vi "Add Subscription.vi"(6 "Notification?(F)":bool, 8 "error in (no error)":errorcluster, 9 "Service Type":T1=4 items=["ONCE_ONLY"=1, "TIMED"=2, "MONITORED"=4], 10 "Subscription Name":string, 11 "DIMActor in":refnum<class "DIMActor.lvclass">) -> (0 "error out":errorcluster, 3 "DIMActor out":refnum<class "DIMActor.lvclass">)   [LabVIEW 2012, in "DIMActor.lvlib" / "DIMActor.lvclass"]
doc: "Subscribe to a DIM service."
uses:
  DIMActor.lvclass
  SVN/LV2009/GPL/lib.lib/DimLVEvent/LVDimInterface/LVDimInterface.dim service type.ctl
  DIMActor.lvclass/DIMActor.ctl
  SVN/LV2009/GPL/lib.lib/DimLVEvent/LVDimInterface/LVDimInterface.dic_info_service_notifier.vi
  SVN/LV2009/GPL/lib.lib/DimLVEvent/LVDimInterface/LVDimInterface.dic_info_service_queue.vi
  SVN/LV2009/GPL/lib.lib/DimLVEvent/LVDimInterface/LVDimInterface.lvlib
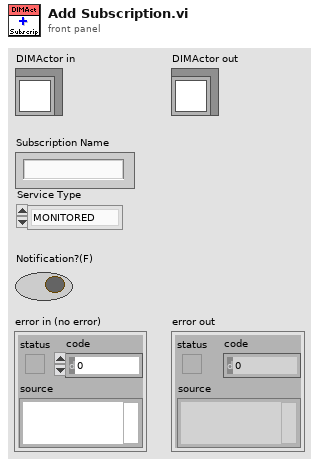
[diagram p1: front panel]
types:
  T1 = typedef "LVDimInterface.lvlib/LVDimInterface.dim service type.ctl" = u16
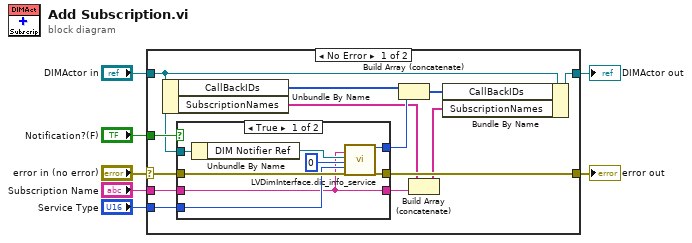
[diagram p0: block diagram]
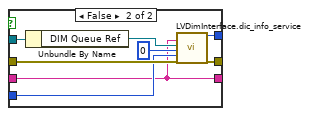
[diagram p2: hidden frame]
diagram:
  n1 = case shown="No Error" "error in (no error)" {
    selector: "error in (no error)" -> [w20 w38]
    tunnel: [w19 w38] -> w6
    tunnel: [w12 w37] -> w4
    tunnel: "DIMActor in" -> [w13 w37]
    tunnel: "Subscription Name" -> [w18 _]
    tunnel: "Notification?(F)" -> [w14 _]
    tunnel: "Service Type" -> [w8 _]
    frame No Error {
      n2 = Unbundle By Name(w13) -> ("CallBackIDs"=w15:i32[], "SubscriptionNames"=w11:string[])
      n3 = case shown="True" w14 {
        tunnel: w20 -> [w25 w33]
        tunnel: [w24 w32] -> w19
        tunnel: w18 -> [w21 w29]
        tunnel: [w26 w34] -> w17
        tunnel: w13 -> [w28 w36]
        tunnel: [w21 w29] -> w10
        tunnel: w8 -> [w22 w30]
        frame True {
          n4 = Unbundle By Name(w28) -> ("DIM Notifier Ref"=w27:refnum<notifier>)
          n5 = call-poly "LVDimInterface.dic_info_service.vi"("serviceName"=w21, "notifierRef"=w27, "timeout [s]"=0, "serviceType"=w22, "error in (no error)"=w25) -> ("callBackID"=w26:i32, "error out"=w24:errorcluster)  [unwired: 13 in]
        }
        frame False {
          n6 = Unbundle By Name(w36) -> ("DIM Queue Ref"=w35:refnum<queue>)
          n7 = call-poly "LVDimInterface.dic_info_service.vi"("serviceName"=w29, "queueRef"=w35, "timeout [s]"=0, "serviceType"=w30, "error in (no error)"=w33) -> ("callBackID"=w34:i32, "error out"=w32:errorcluster)  [unwired: 13 in]
        }
      }
      n8 = Build Array (concatenate)(w15, w17) -> (w16:i32[])
      n9 = Build Array (concatenate)(w11, w10) -> (w9:string[])
      n10 = Bundle By Name(cluster=w13, "CallBackIDs"=w16, "SubscriptionNames"=w9) -> (w12:refnum<class "DIMActor.lvclass">)
    }
    frame Error {
    }
  }
  "error out" <- w6
  "DIMActor out" <- w4
